vi "Full Profiler tester.vi"() -> ()   [LabVIEW 2014]
uses:
  Max profiles.ctl
panel:
  in  "Current Location":dbl(knob) scale=0.0..45.0
  in  "Seconds to graph":dbl=10.0 format="%#_13g"
  in  "Max profiles":T1={"Max jerk"=150.0, "Max acceleration"=20.0, "Max Velocity"=20.0}
  in  "stop":bool
  out "Acceleration Graph 3":cluster{"X":dbl, "Y":dbl}[](graph)
  out "Velocity Graph 2":cluster{"X":dbl, "Y":dbl}[](graph)
  out "Position Graph":cluster{"X":dbl, "Y":dbl}[](graph)
  in  "Setpoint":dbl(knob) scale=0.0..45.0
  out "Motion Profiler Setpoint output":dbl
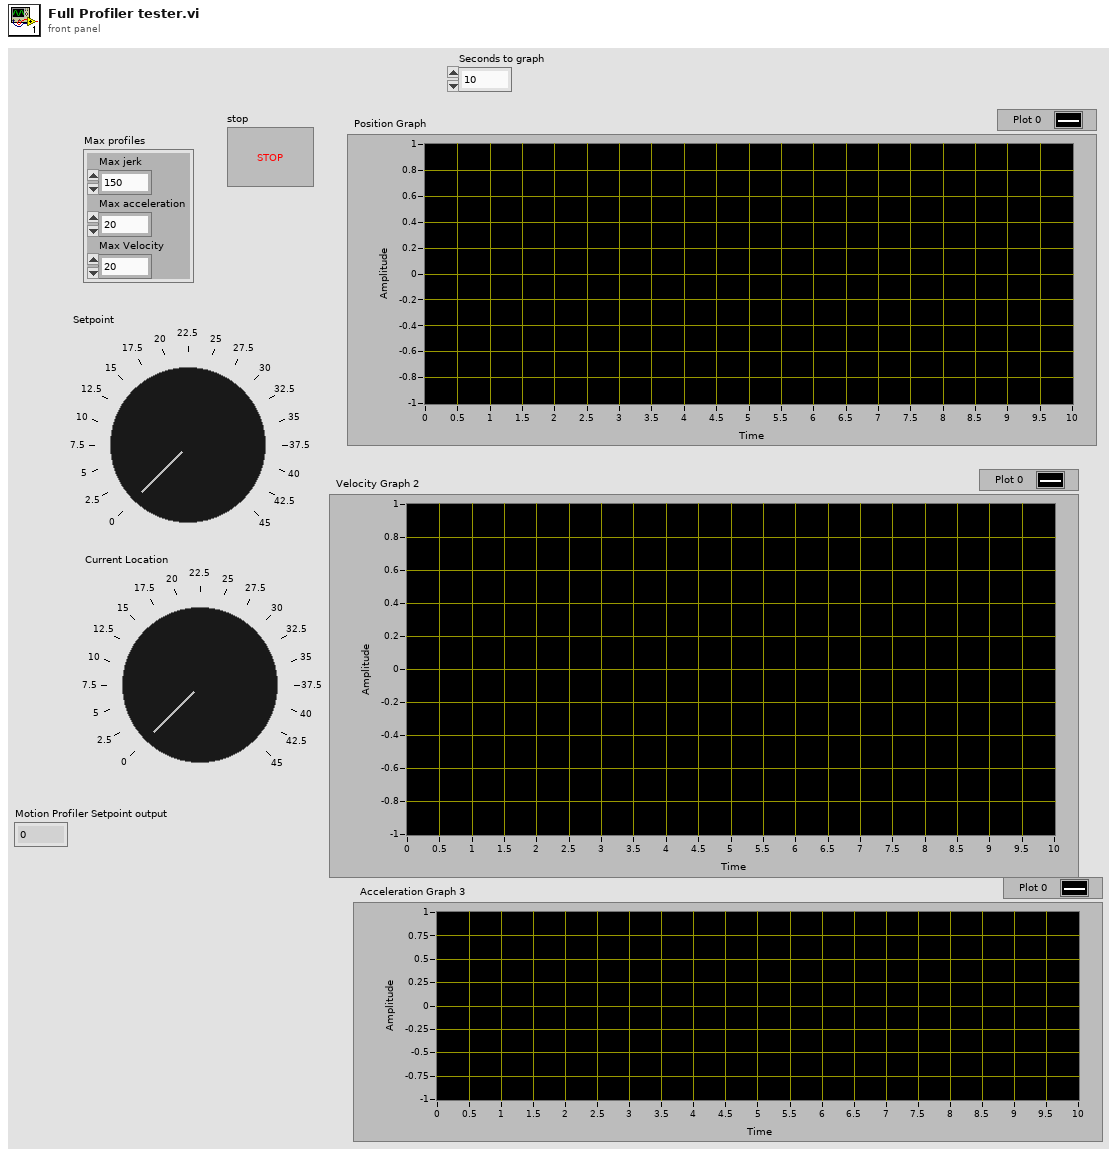
[diagram p1: front panel]
types:
  T1 = typedef "Max profiles.ctl" = cluster{"Max jerk":dbl, "Max acceleration":dbl, "Max Velocity":dbl}
  T2 = typedef "Profiler Shift.ctl" = cluster{"TimeSegments":T3, "Current Setpoint":dbl, "Location at last setpoint change":dbl, "Time at last setpoint change":dbl, "Last Position setpoint":dbl, "Disable Profiler?":bool, "Time at last run":dbl, "Position at last call":dbl}
  T3 = typedef "TimeSegments.ctl" = cluster{"TimeSegments":T4[], "inital velocity":dbl, "inital acceleration":dbl}
  T4 = typedef "TimeSegment.ctl" = cluster{"StartTime":dbl, "TimePeriod":dbl, "PositionAtEnd":dbl, "VelocityAtEnd":dbl}
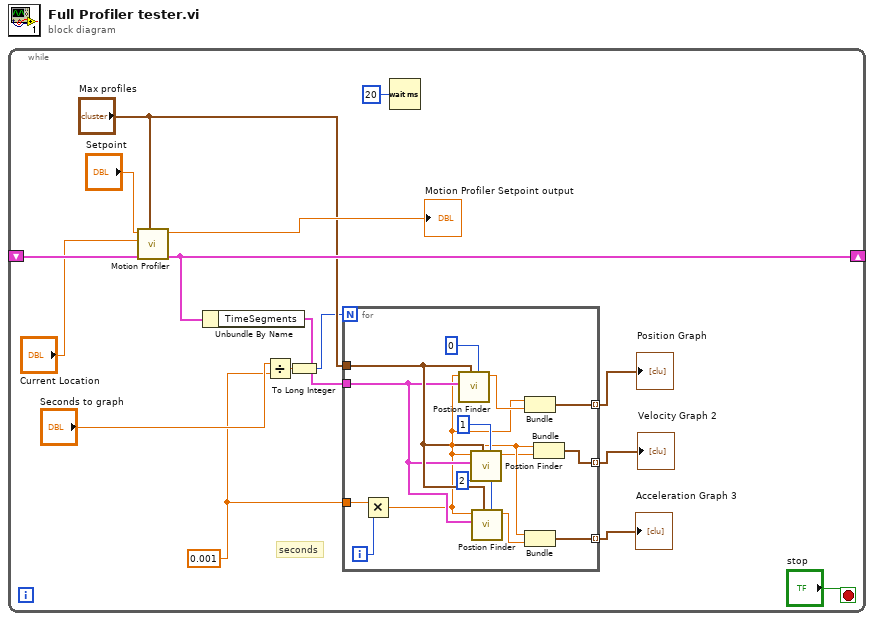
[diagram p0: block diagram]
diagram:
  n1 = while {
    shift-right: [w8] -> _
    shift-left: _ -> [w15]
    stop <- "stop" stop-if-true
    w4 = 0.001
    # "seconds"
    n2 = call "Motion Profiler.vi"("Max profiles"="Max profiles", "From shift"=w15, "Current Location"="Current Location", "Setpoint"="Setpoint") -> ("To Shift"=w8:T2, "Motion Profiler Setpoint output"=→"Motion Profiler Setpoint output":dbl)  [unwired: 6 in]
    n3 = Unbundle By Name(w8) -> ("TimeSegments"=w7:T3)
    n4 = Divide(x="Seconds to graph", y=w4) -> (x/y=w3:dbl)
    n5 = To Long Integer(number=w3) -> (32bit integer=w2:i32)
    n6 = for {
      N: w2 -> [_]
      tunnel: w7 -> [w23]
      tunnel: [w29] -> w10 mode=indexing
      tunnel: "Max profiles" -> [w24]
      tunnel: w4 -> [w28]
      tunnel: [w19] -> w11 mode=indexing
      tunnel: [w18] -> w12 mode=indexing
      i -> [w30]
      n7 = Multiply(x=w28, y=w30) -> (x*y=w21:dbl)
      n8 = call "Postion Finder.vi"("derivitave"=i8 0, "Max profiles"=w24, "TimeSegments"=w23, "time"=w21) -> ("Motion Profiler Setpoint"=w27:dbl)  [unwired: 7 in]
      n9 = call "Postion Finder.vi"("derivitave"=i8 1, "Max profiles"=w24, "TimeSegments"=w23, "time"=w21) -> ("Motion Profiler Setpoint"=w20:dbl)  [unwired: 7 in]
      n10 = call "Postion Finder.vi"("derivitave"=i8 2, "Max profiles"=w24, "TimeSegments"=w23, "time"=w21) -> ("Motion Profiler Setpoint"=w17:dbl)  [unwired: 7 in]
      n11 = Bundle(w21, "Motion Profiler Setpoint"=w27) -> (w29:cluster{dbl, "Motion Profiler Setpoint":dbl})  [unwired: 1 in]
      n12 = Bundle(w21, "Motion Profiler Setpoint"=w17) -> (w18:cluster{dbl, "Motion Profiler Setpoint":dbl})  [unwired: 1 in]
      n13 = Bundle(w21, "Motion Profiler Setpoint"=w20) -> (w19:cluster{dbl, "Motion Profiler Setpoint":dbl})  [unwired: 1 in]
    }
    "Position Graph" <- w10
    "Velocity Graph 2" <- w11
    "Acceleration Graph 3" <- w12
    n14 = Wait (ms)(milliseconds to wait=u32 20) -> ()  [unwired: 1 out]
  }
